vi "Populate Attribute Variant.vi"(8 "error in (no error)":errorcluster, 10 "Property Names":string[](array[string]), 11 "Property Values":variant[](array[variant])) -> (0 "error out":errorcluster, 3 "Attribute Variant out":refnum<class "Variant.lvclass">)   [LabVIEW 2020, in "TDMS.lvlib"]
doc: "Wrap 'Property Values' in generic classes and add them as attributes by 'Property Names' to a generic Variant class."
uses:
  TDMS.lvlib
  PPL/HDH.Data.Generic.lvlibp/Generic Data/Variant/Variant.lvclass
  PPL/HDH.Data.Generic.lvlibp
  PPL/HDH.Data.Generic.lvlibp/Generic Data/Generic Data.lvclass
  C:/Current projects/WS/PPL/HDH.Data.Generic.lvlibp/Data.lvclass
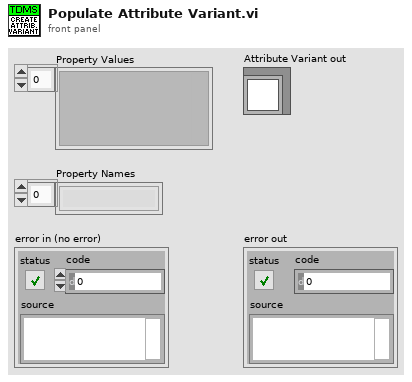
[diagram p1: front panel]
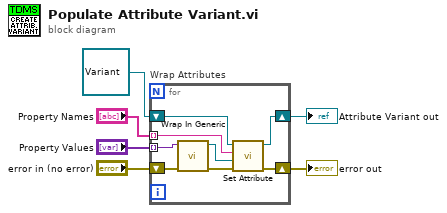
[diagram p0: block diagram]
diagram:
  n1 = for "Wrap Attributes" {
    tunnel: "Property Values" -> [w14] mode=indexing
    tunnel: "Property Names" -> [w11] mode=indexing
    shift-right: [w9] -> w3
    shift-left: refnum<class "Variant.lvclass"> refnum ("HDH.Data.Generic.lvlibp:Variant.lvclass") -> [w13]
    shift-right: [w7] -> w5
    shift-left: "error in (no error)" -> [w8]
    n2 = call "Wrap In Generic.vi"("error in (no error)"=w8, "Data to Wrap"=w14) -> ("error out"=w10:errorcluster, "Generic Data"=w12:refnum<class "Generic Data.lvclass">)  [unwired: 8 in]
    n3 = call "Set Attribute.vi"("error in (no error)"=w10, "Data to set"=w12, "Name"=w11, "Variant in"=w13) -> ("error out"=w7:errorcluster, "Variant out"=w9:refnum<class "Variant.lvclass">)  [unwired: 5 in, 1 out]
  }
  "error out" <- w5
  "Attribute Variant out" <- w3
